vi "ODH_LEGO_Programatically_Close_Consumer.vi"(8 "Error In":errorcluster, 11 "vi path":path=path "D:/Licenta/LEGO_Comfort_Close_Sensor_Activation.vi") -> (0 "Error Out":errorcluster)   [LabVIEW 2016]
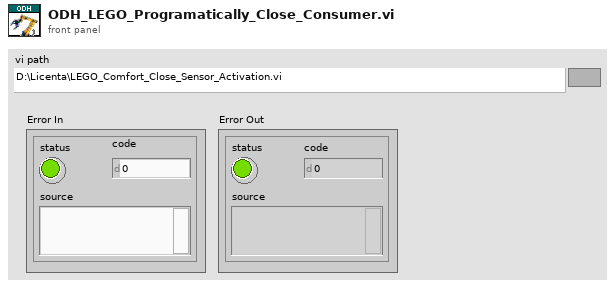
[diagram p1: front panel]
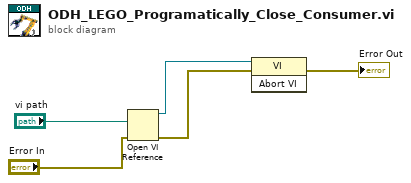
[diagram p0: block diagram]
diagram:
  n1 = Open VI Reference(vi path="vi path", error in (no error)="Error In") -> (vi reference=w4:refnum<vi>, error out=w3:errorcluster)  [unwired: 4 in]
  n2 = invoke class="VI" method="Abort VI"(reference=w4, error in=w3) -> (error out=→"Error Out":errorcluster)  [unwired: 1 in, 2 out]
